vi "Constructor.vi"(5 "TimeZoneInfoId":string, 6 "MeasureExecutionStatus":T1=enum."NOT_COMPLETED", 7 "MeasureTime":timestamp, 8 "error in":errorcluster, 9 "Precision (6)":u8=6, 10 "Value":dbl, 11 "Name":string) -> (0 "error out":errorcluster, 3 "RealMeasure":refnum<class "RealMeasure.lvclass">)   [LabVIEW 2021, in "ProligentXMLGenerator.lvlib" / "RealMeasure.lvclass"]
uses:
  RealMeasure.lvclass
  RealMeasure.lvclass/RealMeasure.ctl
  Measure/Measure.lvclass
  Base/MeasureKind/Value.ctl
  Base/MeasureKind/MeasureKind.lvclass
  Base/UnsignedByte/UnsignedByte.lvclass
  Data.ctl
  Base/Decimal/Decimal.lvclass
  C:/Projects/proligent-xml-generator-labview/src/ProligentXMLGenerator/Measure/Measure/Measure.lvclass
  C:/Projects/proligent-xml-generator-labview/src/ProligentXMLGenerator/Measure/RealMeasure/RealMeasure.lvclass
  Base/ExecutionStatus/Value.ctl
  Base/ExecutionStatus/ExecutionStatus.lvclass
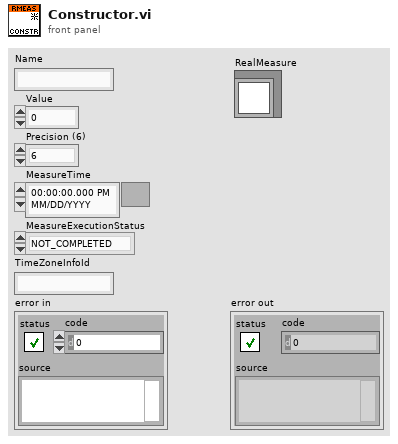
[diagram p1: front panel]
types:
  T1 = typedef "ProligentXMLGenerator.lvlib/ExecutionStatus.lvclass/Value.ctl" = enum16{"PASS", "FAIL", "NOT_COMPLETED", "ABORTED"}
  T2 = typedef "ProligentXMLGenerator.lvlib/RealMeasure.lvclass/Data.ctl" = cluster{"Value":refnum<class "Decimal.lvclass">, "Precision":refnum<class "UnsignedByte.lvclass">}
  T3 = typedef "ProligentXMLGenerator.lvlib/MeasureKind.lvclass/Value.ctl" = enum16{"REAL", "BOOL", "INTEGER", "STRING", "DATETIME"}
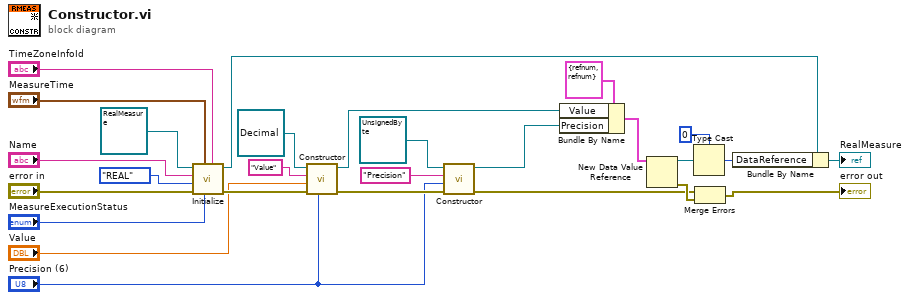
[diagram p0: block diagram]
diagram:
  n1 = call "Initialize.vi"("TimeZoneInfoId"="TimeZoneInfoId", "MeasureExecutionStatus"="MeasureExecutionStatus", "MeasureTime"="MeasureTime", "error in"="error in", "Type"=Value."REAL", "Name"="Name", "Measure in"=refnum<class "RealMeasure.lvclass"> refnum ("ProligentResultProcessor:RealMeasure")) -> ("error out"=w8:errorcluster, "Measure out"=w19:refnum<class "RealMeasure.lvclass">)  [unwired: 3 in]
  n2 = call-dynamic "Constructor.vi"("Precision"="Precision (6)", "error in"=w8, "Value"="Value", "Name"="Value", "Decimal in"=refnum<class "Decimal.lvclass"> refnum ("ProligentResultProcessor:Decimal")) -> ("error out"=w7:errorcluster, "Decimal out"=w3:refnum<class "Decimal.lvclass">)  [unwired: 5 in]
  n3 = call-dynamic "Constructor.vi"("error in"=w7, "Value"="Precision (6)", "Name"="Precision", "UnsignedByte in"=refnum<class "UnsignedByte.lvclass"> refnum ("ProligentResultProcessor:UnsignedByte")) -> ("error out"=w2:errorcluster, "UnsignedByte out"=w20:refnum<class "UnsignedByte.lvclass">)  [unwired: 6 in]
  n4 = Bundle By Name(cluster=T2 {"Value"=refnum, "Precision"=refnum} ("Data"), "Value"=w3, "Precision"=w20) -> (w13:T2)
  n5 = New Data Value Reference(data value=w13) -> (data value reference=w21:refnum<data-value>, error out=w24:errorcluster)  [unwired: 1 in]
  n6 = Type Cast(type=u64 0, x=w21) -> (*(type *) &x=w23:u64)
  n7 = Merge Errors(w2, w24) -> (→"error out":errorcluster)
  n8 = Bundle By Name(cluster=w19, "DataReference"=w23) -> (→"RealMeasure":refnum<class "RealMeasure.lvclass">)
